vi "DronePhotoAndMove.vi"() -> ()   [LabVIEW 2017]
uses:
  <vilib>/LVH/AR Drone Toolkit/Decode NavData/Typedefs/NavData Demo.ctl
  <vilib>/LVH/AR Drone Toolkit/AR Drone.lvlib
panel:
  out "Control cluster":T1 {"Roll" scale=-1.0..1.0; "Pitch" scale=-1.0..1.0; "Vertical Speed" scale=-1.0..1.0; "Yaw Speed" scale=-1.0..1.0}
  out "Python server reply":string
  out "unsigned byte array":u8[](array[numeric])
  in  "stop":bool
  in  "Take Photos":bool
  out "Photos Taken":dbl
  in  "Setup Parameters":T2={"Drone IP address"="192.168.1.1", "Home IP address"="192.168.1.2", "Flight Mode"=enum."INDOOR MODE", "Mounted Hull"=enum."INDOOR HULL", "Video Camera"=0, "Max Altitude (m)"=3.0, "Max Pitch and Roll Angle (deg)"=10.0, "Max Vertical Speed (m/s)"=0.7, "Max Yaw Speed (deg/s)"=100.0} {"Video Camera" items=["Bottom Camera"=1, "Front Camera"=0, "Front in Bottom"=3, "Bottom in Front"=2]}
  out "Video Stream":picture
  out "NavData Out":T3
  out "Battery Remaining":dbl(slide) scale=0.0..100.0
  in  "Hover":bool
  in  "Take Off/Land":bool
  in  "Emergency Landing":bool
  in  "stop 2":bool
  in  "Control Cluster":T4 {"Yaw Speed" scale=-1.0..1.0; "Vertical Speed" scale=-1.0..1.0; "Pitch" scale=-1.0..1.0; "Roll" scale=-1.0..1.0}
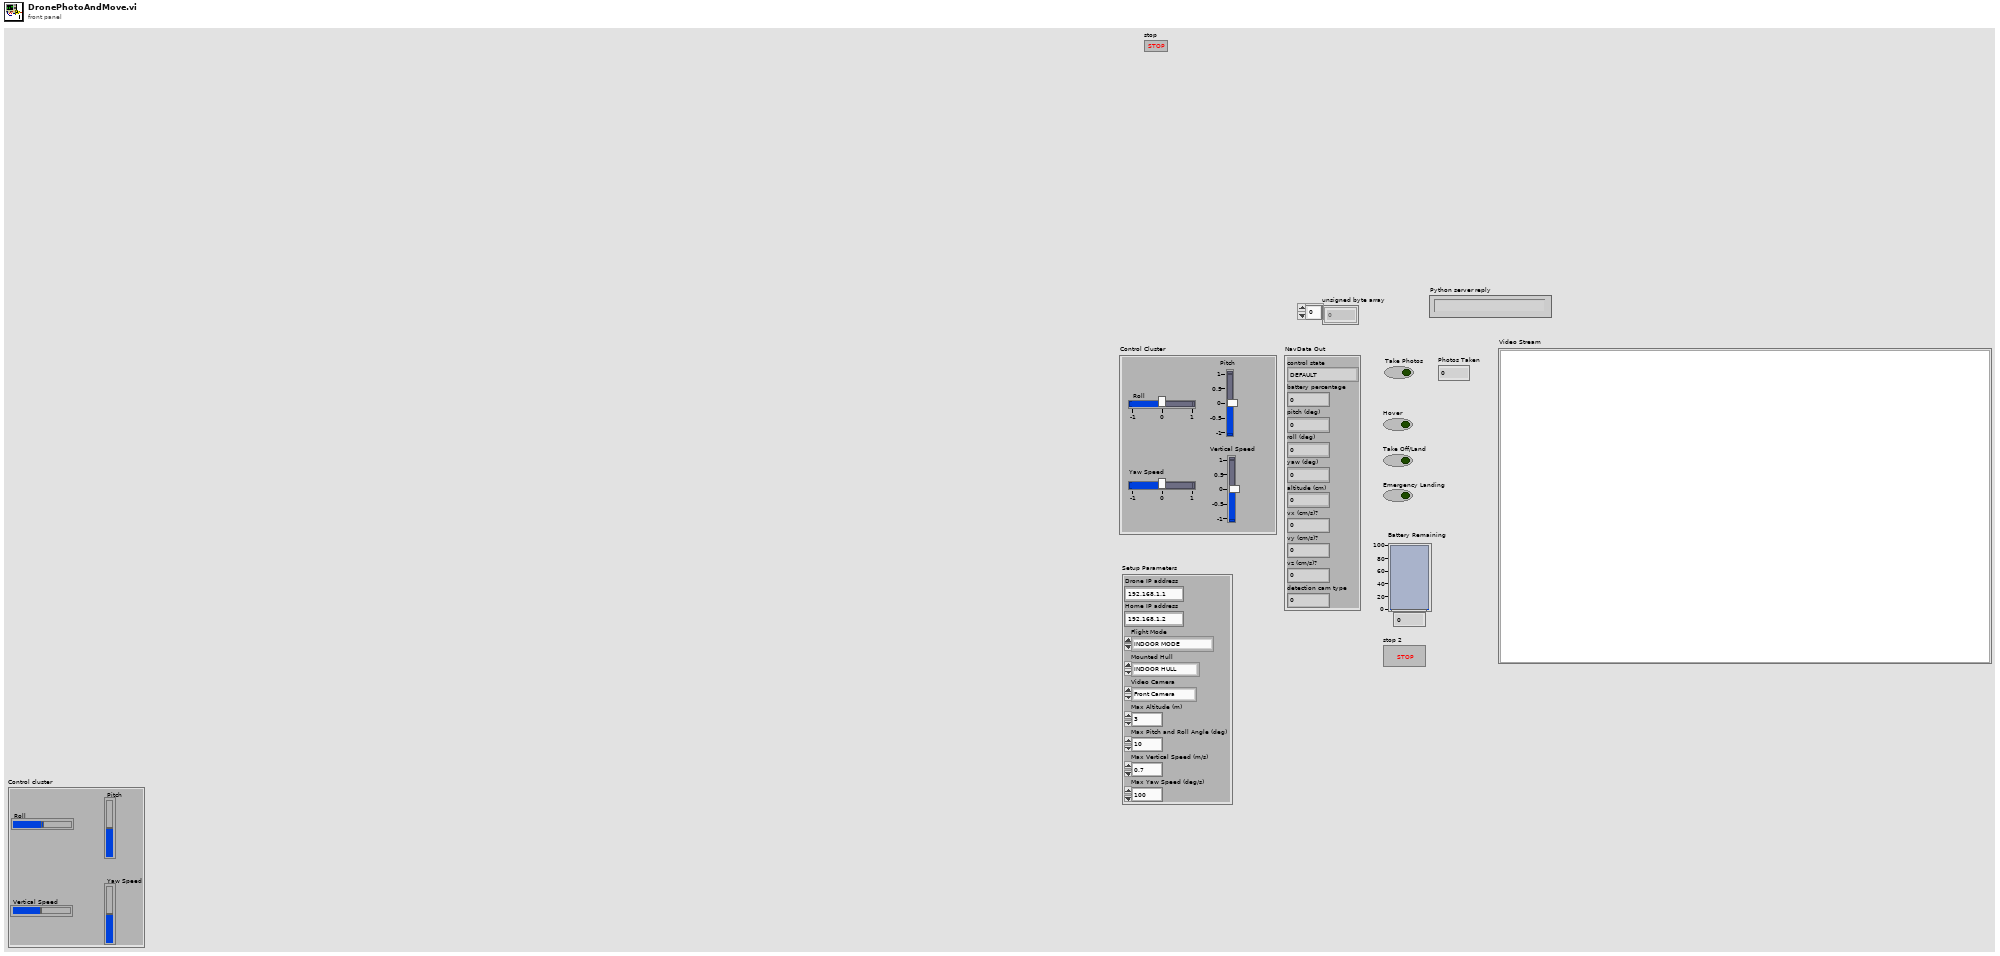
[diagram p1: front panel]
types:
  T1 = cluster{"Roll":dbl, "Pitch":dbl, "Vertical Speed":dbl, "Yaw Speed":dbl}
  T2 = cluster{"Drone IP address":string, "Home IP address":string, "Flight Mode":enum8{"OUTDOOR MODE", "INDOOR MODE"}, "Mounted Hull":enum8{"OUTDOOR HULL", "INDOOR HULL"}, "Video Camera":u8, "Max Altitude (m)":sgl, "Max Pitch and Roll Angle (deg)":sgl, "Max Vertical Speed (m/s)":sgl, "Max Yaw Speed (deg/s)":sgl}
  T3 = typedef "AR Drone.lvlib/NavData Demo.ctl" = cluster{"control state":enum32{"DEFAULT", "INIT", "LANDING", "FLYING", "HOVERING", "TEST", "TRANS_TAKEOFF", "TRANS_GOTOFIX", "TRANS_LANDING"}, "battery percentage":u32, "pitch (deg)":sgl, "roll (deg)":sgl, "yaw (deg)":sgl, "altitude (cm)":u32, "vx (cm/s)?":sgl, "vy (cm/s)?":sgl, "vz (cm/s)?":sgl, "detection cam type":u32}
  T4 = cluster{"Roll":sgl, "Pitch":sgl, "Vertical Speed":sgl, "Yaw Speed":sgl}
  T5 = typedef "AR Drone.lvlib/AR Drone Resource.ctl" = cluster{"UDP Control Connection":refnum<k16>, "UDP NavData Connection":refnum<k16>, "UDP Video Connection (Drone 1.0)":refnum<k16>, "TCP Video Connection (Drone 2.0)":refnum<k5>, "TCP Control Port Connection":refnum<k5>, "Drone IP address":string, "Drone Command Port":u16, "Drone NavData Port":u16, "Drone Vid Stream Port":u16, "Drone TCP Control Port":u16, "Home IP address":string, "Home Command Port":u16, "Home NavData Port":u16, "Home Vid Stream Port":u16, "Drone Version":i32, "Drone Index":dbl}
  T6 = cluster{"Boolean array[0]":bool, "Boolean array[1]":bool, "Boolean array[2]":bool, "Boolean array[3]":bool, "Boolean array[4]":bool, "Boolean array[5]":bool, "Boolean array[6]":bool, "Boolean array[7]":bool, "Boolean array[8]":bool}
  T7 = typedef "IMAQ Image.ctl" = refnum<image>
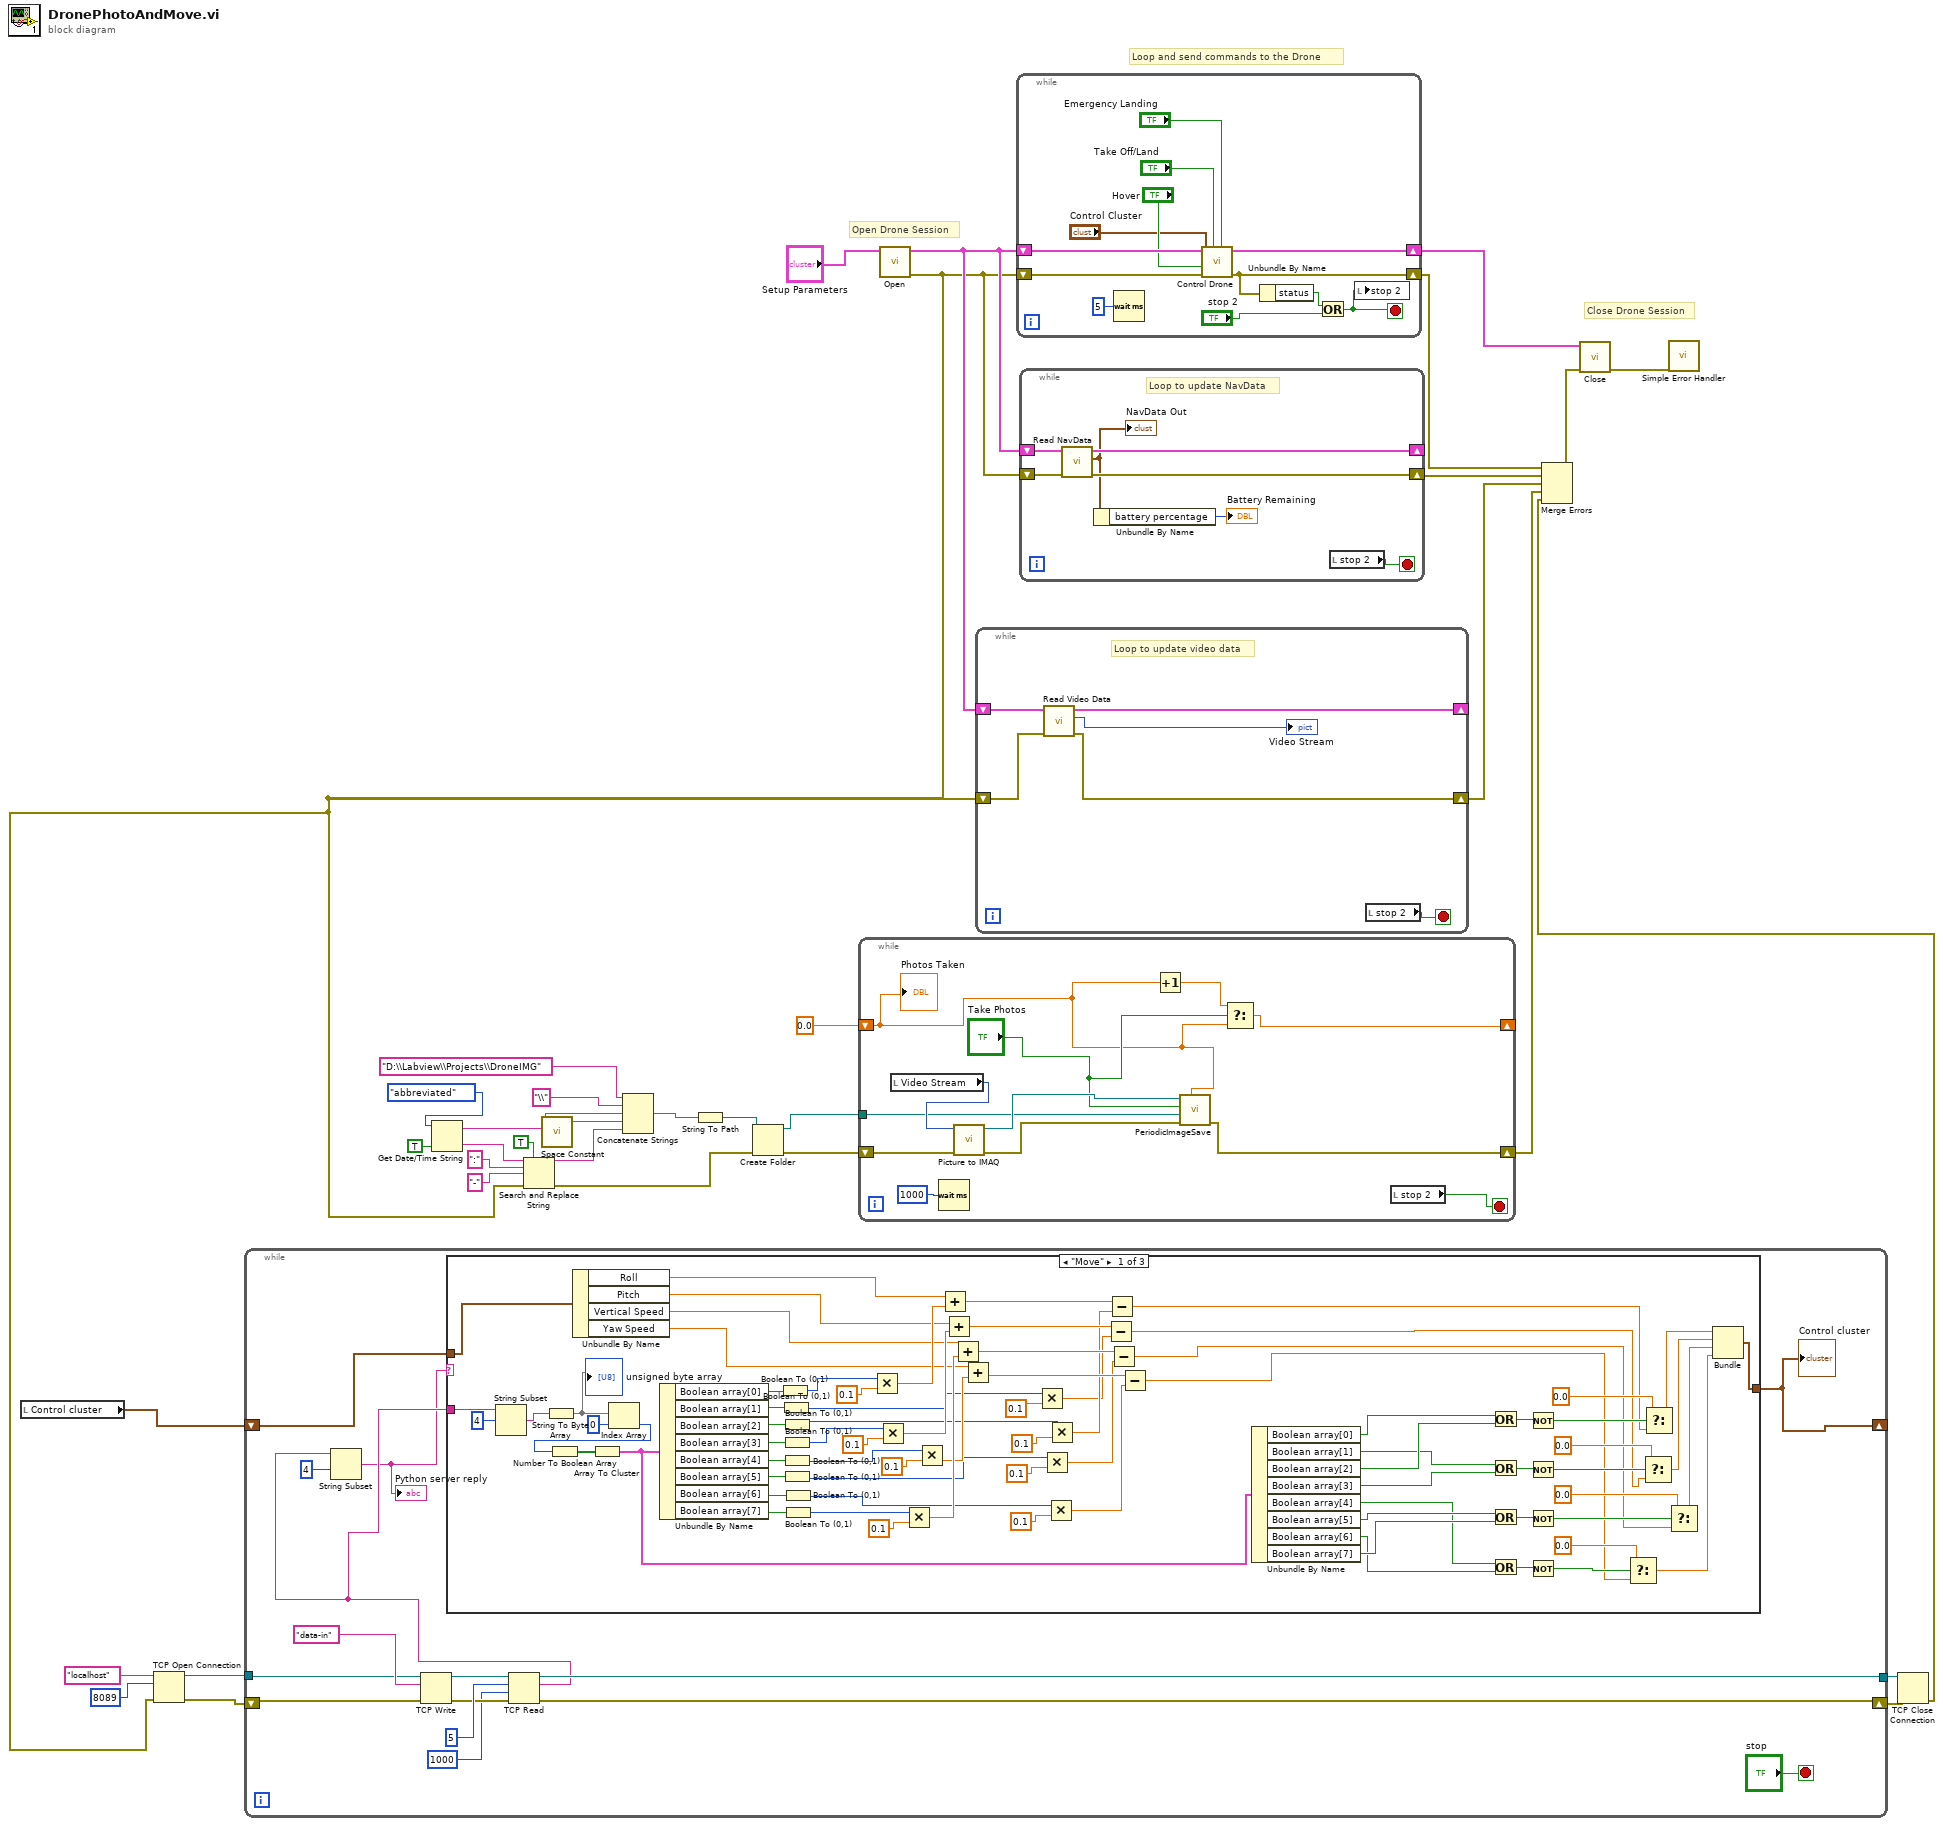
[diagram p0: block diagram]
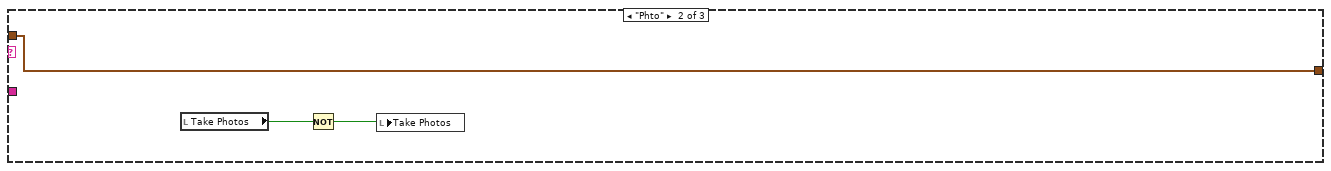
[diagram p2: hidden frame]
diagram:
  # "Close Drone Session"
  # "Loop and send commands to the Drone"
  # "Open Drone Session"
  n1 = local read "Control cluster"() -> (w1:T1)
  n2 = Get Date/Time String(date format (0)=enum16{"short", "long", "abbreviated"}."abbreviated", want seconds? (F)=TRUE) -> (date string=w25:string, time string=w22:string)  [unwired: 1 in]
  n3 = call <vilib>:"Space Constant.vi"() -> ("String"=w24:string)
  n4 = call <vilib>:"Open.vi"("Setup Parameters"="Setup Parameters") -> ("error out"=w5:errorcluster, "AR Drone Resource"=w33:T5)  [unwired: 9 in]
  n5 = TCP Open Connection(address="localhost", remote port or service name=u16 8089, error in (no error)=w5) -> (connection ID=w6:refnum<k5>, error out=w2:errorcluster)  [unwired: 2 in]
  n6 = while {
    tunnel: [w44] -> w9
    tunnel: w6 -> [w43]
    shift-right: [w36] -> _
    shift-left: w1 -> [w41]
    shift-right: [w39] -> w3
    shift-left: w2 -> [w38]
    stop <- "stop" stop-if-true
    n7 = TCP Write(connection ID=w43, data in="data-in", error in (no error)=w38) -> (connection ID out=w49:refnum<k5>, error out=w48:errorcluster)  [unwired: 1 in, 1 out]
    n8 = TCP Read(connection ID=w49, bytes to read=5, error in (no error)=w48, 9:1000 ("timeout ms (25000)")) -> (connection ID out=w44:refnum<k5>, data out=w40:string, error out=w39:errorcluster)  [unwired: 1 in]
    n9 = String Subset(string=w40, length (rest)=4 ("length (rest)")) -> (substring=w37:string)  [unwired: 1 in]
    "Python server reply" <- w37
    n10 = case shown="\"Move\"" w37 {
      tunnel: [w124 w130 w132] -> w36
      tunnel: w41 -> [w51 w130 w132]
      tunnel: w40 -> [w128 _ _]
      frame "Move" {
        n11 = String Subset(string=w128, offset (0)=4) -> (substring=w126:string)  [unwired: 1 in]
        n12 = String To Byte Array(string=w126) -> (unsigned byte array=w56:u8[])
        "unsigned byte array" <- w56
        n13 = Unbundle By Name(w51) -> ("Roll"=w55:dbl, "Pitch"=w54:dbl, "Vertical Speed"=w53:dbl, "Yaw Speed"=w52:dbl)
        n14 = Index Array(array=w56, index=0) -> (element=w110:u8)
        n15 = Number To Boolean Array(number=w110) -> (Boolean array=w123:bool[])
        n16 = Array To Cluster(array=w123) -> (cluster=w73:T6)
        n17 = Unbundle By Name(w73) -> ("Boolean array[0]"=w118:bool, "Boolean array[1]"=w117:bool, "Boolean array[2]"=w116:bool, "Boolean array[3]"=w115:bool, "Boolean array[4]"=w114:bool, "Boolean array[5]"=w113:bool, "Boolean array[6]"=w112:bool, "Boolean array[7]"=w111:bool)
        n18 = Boolean To (0,1)(Boolean=w118) -> (0, 1=w98:i16)
        n19 = Boolean To (0,1)(Boolean=w117) -> (0, 1=w87:i16)
        n20 = Boolean To (0,1)(Boolean=w116) -> (0, 1=w89:i16)
        n21 = Boolean To (0,1)(Boolean=w115) -> (0, 1=w102:i16)
        n22 = Boolean To (0,1)(Boolean=w114) -> (0, 1=w101:i16)
        n23 = Boolean To (0,1)(Boolean=w113) -> (0, 1=w93:i16)
        n24 = Boolean To (0,1)(Boolean=w112) -> (0, 1=w96:i16)
        n25 = Boolean To (0,1)(Boolean=w111) -> (0, 1=w108:i16)
        n26 = Multiply(x=w98, y=0.1) -> (x*y=w99:dbl)
        n27 = Multiply(x=w102, y=0.1) -> (x*y=w103:dbl)
        n28 = Multiply(x=w108, y=0.1) -> (x*y=w107:dbl)
        n29 = Multiply(x=w101, y=0.1) -> (x*y=w105:dbl)
        n30 = Add(x=w55, y=w99) -> (x+y=w122:dbl)
        n31 = Add(x=w54, y=w103) -> (x+y=w121:dbl)
        n32 = Add(x=w53, y=w107) -> (x+y=w120:dbl)
        n33 = Add(x=w52, y=w105) -> (x+y=w119:dbl)
        n34 = Multiply(x=w87, y=0.1) -> (x*y=w86:dbl)
        n35 = Multiply(x=w93, y=0.1) -> (x*y=w92:dbl)
        n36 = Multiply(x=w96, y=0.1) -> (x*y=w95:dbl)
        n37 = Multiply(x=w89, y=0.1) -> (x*y=w88:dbl)
        n38 = Subtract(x=w121, y=w86) -> (x-y=w60:dbl)
        n39 = Subtract(x=w122, y=w88) -> (x-y=w58:dbl)
        n40 = Subtract(x=w120, y=w92) -> (x-y=w62:dbl)
        n41 = Subtract(x=w119, y=w95) -> (x-y=w64:dbl)
        n42 = Unbundle By Name(w73) -> ("Boolean array[0]"=w72:bool, "Boolean array[1]"=w70:bool, "Boolean array[2]"=w71:bool, "Boolean array[3]"=w69:bool, "Boolean array[4]"=w66:bool, "Boolean array[5]"=w67:bool, "Boolean array[6]"=w65:bool, "Boolean array[7]"=w68:bool)
        n43 = Or(x=w72, y=w71) -> (x .or. y?=w85:bool)
        n44 = Or(x=w70, y=w69) -> (x .or. y?=w82:bool)
        n45 = Or(x=w67, y=w68) -> (x .or. y?=w79:bool)
        n46 = Or(x=w66, y=w65) -> (x .or. y?=w76:bool)
        n47 = Not(x=w85) -> (.not. x?=w84:bool)
        n48 = Not(x=w82) -> (.not. x?=w81:bool)
        n49 = Not(x=w79) -> (.not. x?=w78:bool)
        n50 = Not(x=w76) -> (.not. x?=w75:bool)
        n51 = Select(t=0.0, s=w75, f=w64) -> (s? t:f=w63:dbl)
        n52 = Select(t=0.0, s=w81, f=w60) -> (s? t:f=w59:dbl)
        n53 = Select(t=0.0, s=w84, f=w58) -> (s? t:f=w57:dbl)
        n54 = Select(t=0.0, s=w78, f=w62) -> (s? t:f=w61:dbl)
        n55 = Bundle("t"=w57, "t"=w59, "t"=w61, "t"=w63) -> (w124:cluster{"t":dbl, "t":dbl, "t":dbl, "t":dbl})  [unwired: 1 in]
      }
      frame "Phto" {
        n56 = local read "Take Photos"() -> (w129:bool)
        n57 = Not(x=w129) -> (.not. x?=w131:bool)
        n58 = local write "Take Photos"(w131) -> ()
      }
      frame " ", Default {
      }
    }
    "Control cluster" <- w36
  }
  n59 = Search and Replace String(replace all?=TRUE ("replace all? (F)"), input string=w22, search string=":" ("replace string (\"\")"), replace string="-" ("replace string (\"\")"), error in=w5) -> (result string=w23:string, error out=w13:errorcluster)  [unwired: 3 in, 2 out]
  n60 = Concatenate Strings("D:\\Labview\\Projects\\DroneIMG" ("string"), "\\" ("string"), w25, w24, w23) -> (w15:string)
  n61 = String To Path(string=w15) -> (path=w14:path)
  n62 = Create Folder(path (use dialog)=w14, error in=w13) -> (created path=w11:path, error out=w12:errorcluster)  [unwired: 1 in, 1 out]
  n63 = while {
    shift-right: [w134] -> w27
    shift-left: w12 -> [w143]
    shift-right: [w136] -> _
    shift-left: 0.0 -> [w135]
    tunnel: w11 -> [w133]
    stop <- w144 stop-if-true
    n64 = local read "Video Stream"() -> (w142:picture)
    n65 = Wait (ms)(milliseconds to wait=u32 1000) -> ()  [unwired: 1 out]
    n66 = call "Picture to IMAQ.vi"("Error In"=w143, "picture"=w142) -> ("Error Out"=w140:errorcluster, "Image"=w139:T7)  [unwired: 8 in]
    n67 = Increment(x=w135) -> (x+1=w138:dbl)
    n68 = call "PeriodicImageSave.vi"("x"=w135, "error in (no error)"=w140, "in path"=w133, "Snap"="Take Photos", "Image In"=w139) -> ("error out"=w134:errorcluster)  [unwired: 5 in]
    n69 = Select(t=w138, s="Take Photos", f=w135) -> (s? t:f=w136:dbl)
    n70 = local read "stop 2"() -> (w144:bool)
    "Photos Taken" <- w135
  }
  n71 = while {
    shift-right: [w147] -> _
    shift-left: w33 -> [w149]
    shift-right: [w145] -> w28
    shift-left: w5 -> [w148]
    stop <- w150 stop-if-true
    # "Loop to update video data"
    n72 = call <vilib>:"Read Video Data.vi"("error in (no error)"=w148, "AR Drone Resource"=w149) -> ("error out"=w145:errorcluster, "Video Stream"=→"Video Stream":picture, "AR Drone Resource Out"=w147:T5)  [unwired: 7 in]
    n73 = local read "stop 2"() -> (w150:bool)
  }
  n74 = while {
    shift-right: [w157] -> w35
    shift-left: w33 -> [w161]
    shift-right: [w152] -> w30
    shift-left: w5 -> [w162]
    stop <- w151 stop-if-true
    n75 = Wait (ms)(milliseconds to wait=u32 5) -> ()  [unwired: 1 out]
    n76 = call <vilib>:"Control Drone.vi"("Emergency Landing"="Emergency Landing", "Takeoff/Land"="Take Off/Land", "error in (no error)"=w162, "Hover"="Hover", "Control Cluster"="Control Cluster", "AR Drone Resource"=w161) -> ("error out"=w152:errorcluster, "AR Drone Resource Out"=w157:T5)  [unwired: 4 in]
    n77 = Unbundle By Name(w152) -> ("status"=w154:bool)
    n78 = Or(x=w154, y="stop 2") -> (x .or. y?=w151:bool)
    n79 = local write "stop 2"(w151) -> ()
  }
  n80 = while {
    shift-right: [w167] -> _
    shift-left: w33 -> [w168]
    shift-right: [w165] -> w31
    shift-left: w5 -> [w166]
    stop <- w169 stop-if-true
    # "Loop to update NavData"
    n81 = call <vilib>:"Read NavData.vi"("error in (no error)"=w166, "AR Drone Resource"=w168) -> ("error out"=w165:errorcluster, "NavData Out"=w164:T3, "AR Drone Resource Out"=w167:T5)  [unwired: 7 in]
    "NavData Out" <- w164
    n82 = Unbundle By Name(w164) -> ("battery percentage"=→"Battery Remaining":u32)
    n83 = local read "stop 2"() -> (w169:bool)
  }
  n84 = TCP Close Connection(connection ID=w9, error in (no error)=w3) -> (error out=w4:errorcluster)  [unwired: 1 in, 1 out]
  n85 = Merge Errors(w30, w31, w28, w27, w4) -> (w32:errorcluster)
  n86 = call <vilib>:"Close.vi"("error in (no error)"=w32, "AR Drone Resource"=w35) -> ("error out"=w34:errorcluster)  [unwired: 9 in]
  n87 = call <vilib>:"Simple Error Handler.vi"("error in (no error)"=w34) -> ()  [unwired: 4 in, 5 out]
